vi "Initialize Work.vi"(8 "error in (no error)":errorcluster, 9 "Update period":dbl, 10 "Reply to":refnum<class "Result Reply Msg.lvclass">, 11 "Measure Object in":refnum<class "Worker.lvclass">) -> (0 "error out":errorcluster, 3 "Measure Object out":refnum<class "Worker.lvclass">)   [LabVIEW 2018, in "Worker.lvclass"]
uses:
  Worker.lvclass
  C:/github/LabActor/Template Module/Template Module.lvclass
  Template Module Messages/Result Reply Msg/Result Reply Msg.lvclass
  C:/github/LabActor/Template Module Messages/Self-Addressed Msg/Self-addressed Msg.lvclass
  Worker.lvclass/Worker.ctl
  NHMFL_Core/Libraries/Instruments/Instrument Driver/Worker State.ctl
  Template Module/Template Module.lvclass/Template Module.ctl
  NHMFL_Core/Libraries/Instruments/Results/Acquired Result/Acquired Result.lvclass/Acquired Result.ctl
  Template Module Messages/Self-Addressed Msg/Self-addressed Msg.lvclass/Self-addressed Msg.ctl
  Controllers/Process Controller Messages/Stop Measurements Msg/Stop Measurements Msg.lvclass/Stop Measurements Msg.ctl
  <vilib>/ActorFramework/Message Enqueuer/Message Enqueuer.lvclass/Message Enqueuer.ctl
  Template Module/Write State.vi
  Template Module/Read Reply to.vi
  Template Module/Read Name.vi
  NHMFL_Core/Libraries/Instruments/Results/Acquired Result/Write Sender.vi
  Template Module Messages/Self-Addressed Msg/Read Return Enqueuer.vi
  Template Module/Write Reply to.vi
  Write Cycle period.vi
  Write Cycle count.vi
  Write Pause requested.vi
  Write Paused.vi
  Write Done.vi
  Template Module/Read State.vi
  <vilib>/ActorFramework/Message Enqueuer/Enqueue.vi
  Controllers/Process Controller Messages/Stop Measurements Msg/Stop Measurements Msg.lvclass
  C:/Program Files/National Instruments/LabVIEW 2018/vi.lib/ActorFramework/Message/Message.lvclass
  <vilib>/ActorFramework/Message Priority Queue/Priority Enqueue.vi
  <vilib>/ActorFramework/Message Enqueuer/Message Enqueuer.lvclass
  NHMFL_Core/Libraries/Instruments/Results/Acquired Result/Acquired Result.lvclass
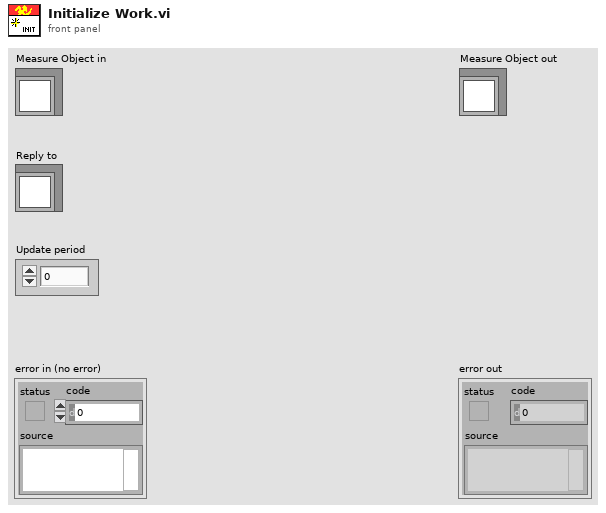
[diagram p1: front panel]
types:
  T1 = typedef "Worker State.ctl" = enum16{"Idle", "Starting", "Working", "Stopping"}
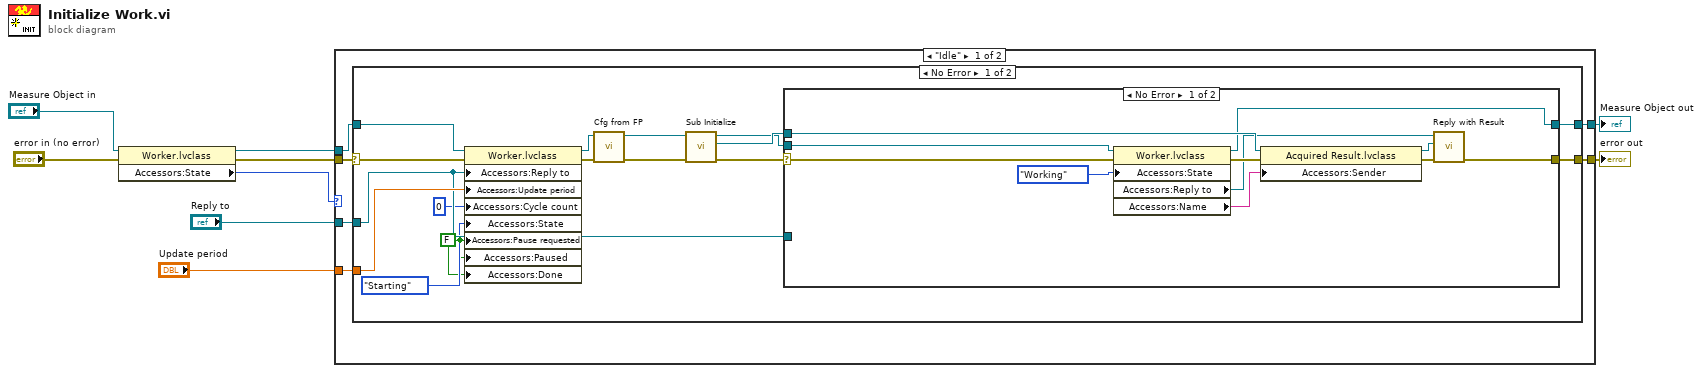
[diagram p0: block diagram]
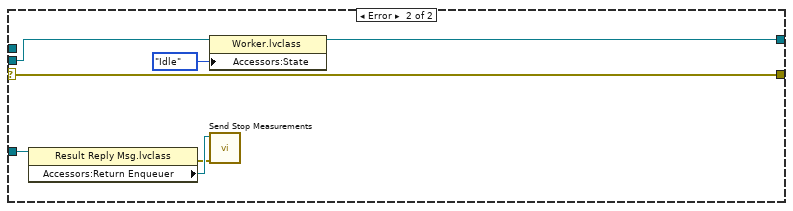
[diagram p2: hidden frame]
diagram:
  n1 = property class="Worker.lvclass"(reference="Measure Object in", error in="error in (no error)") -> (reference out=w4:refnum<class "Worker.lvclass">, error out=w2:errorcluster, "Accessors:State"=w1:T1)
  n2 = case shown="\"Idle\"" w1 {
    tunnel: [w15 w52] -> w9
    tunnel: [w14 w53] -> w8
    tunnel: "Update period" -> [w13 _]
    tunnel: "Reply to" -> [w12 _]
    tunnel: w4 -> [w11 w53]
    tunnel: w2 -> [w10 w52]
    frame "Idle" {
      n3 = case shown="No Error" w10 {
        selector: w10 -> [w25 w51]
        tunnel: [w31 w51] -> w15
        tunnel: [w22 w50] -> w14
        tunnel: w11 -> [w30 w50]
        tunnel: w13 -> [w21 _]
        tunnel: w12 -> [w19 _]
        frame No Error {
          w16 = FALSE ("Pause requested")
          n4 = property class="Worker.lvclass"(reference=w30, error in=w25, "Accessors:Reply to"=w19, "Accessors:Update period"=w21, "Accessors:Cycle count"=0 ("Cycle count"), "Accessors:State"=Worker_State."Starting" ("State"), "Accessors:Pause requested"=w16, "Accessors:Paused"=w16, "Accessors:Done"=w16) -> (reference out=w26:refnum<class "Worker.lvclass">, error out=w24:errorcluster)
          n5 = call-dynamic "Cfg from FP.vi"("error in (no error)"=w24, "Measure Object in"=w26) -> ("error out"=w27:errorcluster, "Measure Object out"=w29:refnum<class "Worker.lvclass">)  [unwired: 8 in]
          n6 = call-dynamic "Sub Initialize.vi"("error in (no error)"=w27, "Measure Object in"=w29) -> ("error out"=w20:errorcluster, "Initialize Result"=w28:refnum<class "Acquired Result.lvclass">, "Measure Object out"=w23:refnum<class "Worker.lvclass">)  [unwired: 7 in]
          n7 = case shown="No Error" w20 {
            selector: w20 -> [w34 w45]
            tunnel: [w42 w45] -> w31
            tunnel: w28 -> [w39 _]
            tunnel: w23 -> [w38 w49]
            tunnel: [w35 w44] -> w22
            tunnel: w19 -> [_ w48]
            frame No Error {
              n8 = property class="Worker.lvclass"(reference=w38, error in=w34, "Accessors:State"=Worker_State."Working" ("State")) -> (reference out=w35:refnum<class "Worker.lvclass">, error out=w36:errorcluster, "Accessors:Reply to"=w33:refnum<class "Result Reply Msg.lvclass">, "Accessors:Name"=w37:string)
              n9 = property class="Acquired Result.lvclass"(reference=w39, error in=w36, "Accessors:Sender"=w37) -> (reference out=w40:refnum<class "Acquired Result.lvclass">, error out=w41:errorcluster)
              n10 = call-dynamic "Reply with Result.vi"("error in (no error)"=w41, "Result"=w40, "Result Reply Msg in"=w33) -> ("error out"=w42:errorcluster)  [unwired: 7 in, 1 out]
            }
            frame Error {
              n11 = property class="Result Reply Msg.lvclass"(reference=w48) -> (error out=w46:errorcluster, "Accessors:Return Enqueuer"=w47:refnum<class "Message Enqueuer.lvclass">)  [unwired: 1 in, 1 out]
              n12 = property class="Worker.lvclass"(reference=w49, "Accessors:State"=Worker_State."Idle" ("State")) -> (reference out=w44:refnum<class "Worker.lvclass">)  [unwired: 1 in, 1 out]
              n13 = call "Send Stop Measurements.vi"("error in (no error)"=w46, "Message Enqueuer"=w47) -> ()  [unwired: 8 in, 2 out]
            }
          }
        }
        frame Error {
        }
      }
    }
    frame "Working", Default {
    }
  }
  "error out" <- w9
  "Measure Object out" <- w8
